vi "Convert Hexadecimal string to a Boolean array.vi"(1 "Hexadecimal String IN":string="abcdef") -> (0 "Boolean Array":bool[][](array[boolean]))   [LabVIEW 2013]
panel:
  # "a"
  # "dim 1 : Char #"
  # "b"
  # "abcd"
  # "c"
  # "dim 2 : Bit #"
  # "d"
  # "0    1    2   3"
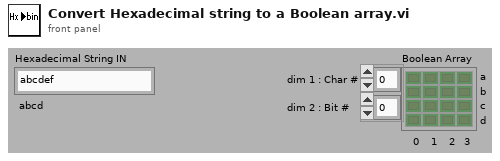
[diagram p1: front panel]
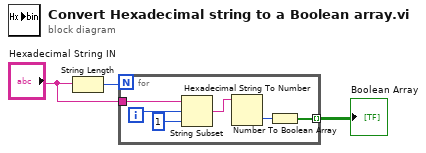
[diagram p0: block diagram]
diagram:
  n1 = String Length(string="Hexadecimal String IN") -> (length=w3:i32)
  n2 = for {
    N: w3 -> [_]
    tunnel: "Hexadecimal String IN" -> [w9]
    tunnel: [w4] -> w1 mode=indexing
    i -> [w8]
    n3 = String Subset(string=w9, offset (0)=w8, length (rest)=1 ("longueur (reste)")) -> (substring=w6:string)
    n4 = Hexadecimal String To Number(string=w6) -> (number=w5:u32)  [unwired: 3 out]
    n5 = Number To Boolean Array(number=w5) -> (Boolean array=w4:bool[])
  }
  "Boolean Array" <- w1
